vi "Mux16.vi"(0 "a":bool[](array[boolean])=[FALSE, FALSE, FALSE, FALSE, FALSE, FALSE, FALSE, FALSE, FALSE, FALSE, FALSE, FALSE, FALSE, FALSE, FALSE, FALSE], 4 "sel":bool, 5 "b":bool[](array[boolean])=[FALSE, FALSE, FALSE, FALSE, FALSE, FALSE, FALSE, FALSE, FALSE, FALSE, FALSE, FALSE, FALSE, FALSE, FALSE, FALSE]) -> (7 "out":bool[](array[boolean]))   [LabVIEW 2014]
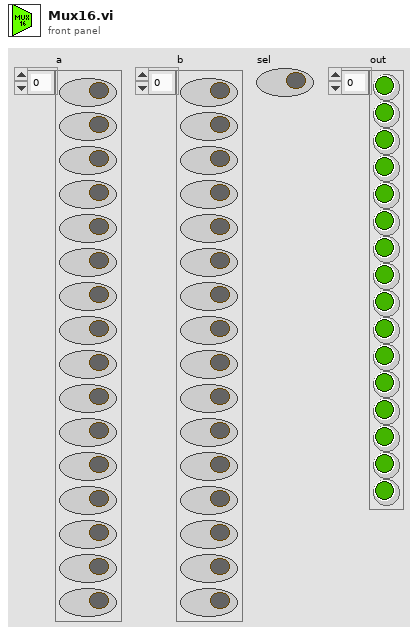
[diagram p1: front panel]
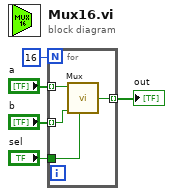
[diagram p0: block diagram]
diagram:
  n1 = for {
    N: 16 -> [_]
    tunnel: "a" -> [w9] mode=indexing
    tunnel: "b" -> [w8] mode=indexing
    tunnel: [w6] -> w2 mode=indexing
    tunnel: "sel" -> [w7]
    n2 = call "Mux.vi"("a"=w9, "sel"=w7, "b"=w8) -> ("out"=w6:bool)  [unwired: 5 in]
  }
  "out" <- w2
